vi "Partially Matched Crossover(PMX).vi"(10 "Ind 2":T1, 11 "Ind 1":T1) -> (2 "Child 2":T1, 3 "Child 1":T1)   [LabVIEW 2013, in "GA.lvclass"]
uses:
  GA.lvclass
  Controls/Solution_GA.ctl
panel:
  out "cxpoint2":i32
  out "cxpoint1":i32
  out "Child2 Schedule":u16[](array[numeric])
  out "Child 1 Schedule":u16[](array[numeric])
  out "p2":i32[](array[numeric])
  out "p1":i32[](array[numeric])
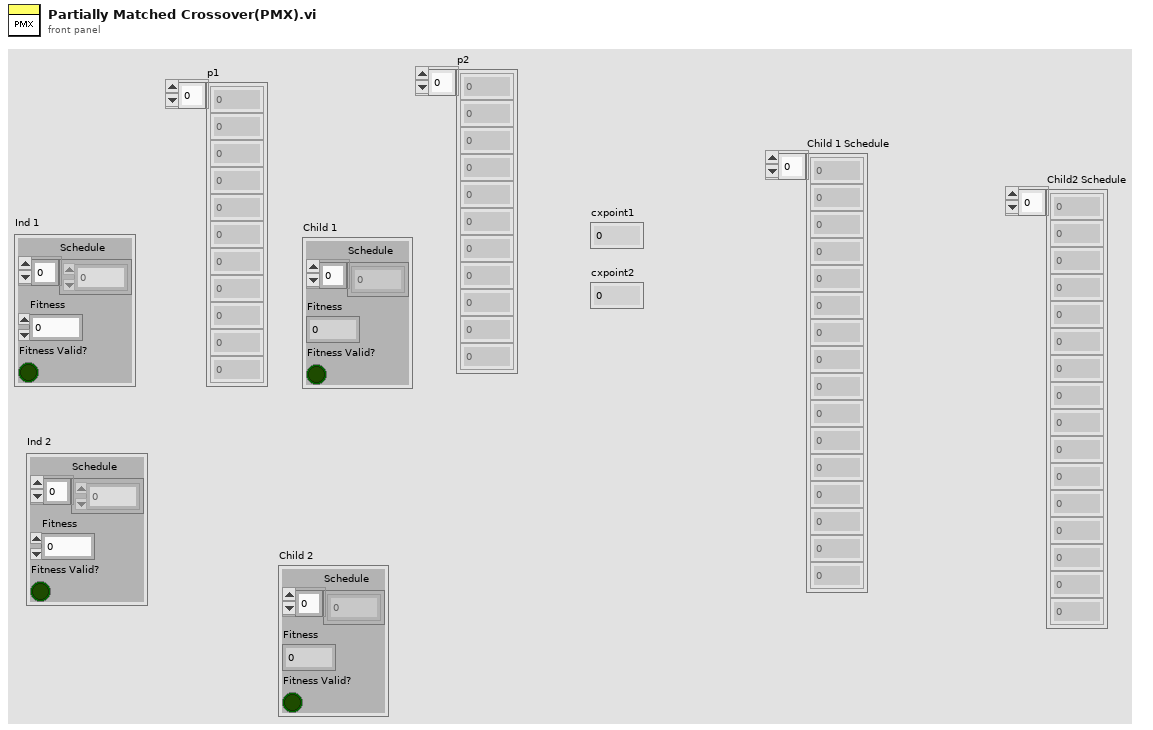
[diagram p1: front panel]
types:
  T1 = typedef "Solution_GA.ctl" = cluster{"Schedule":u16[], "Fitness":u16, "Fitness Valid?":bool}
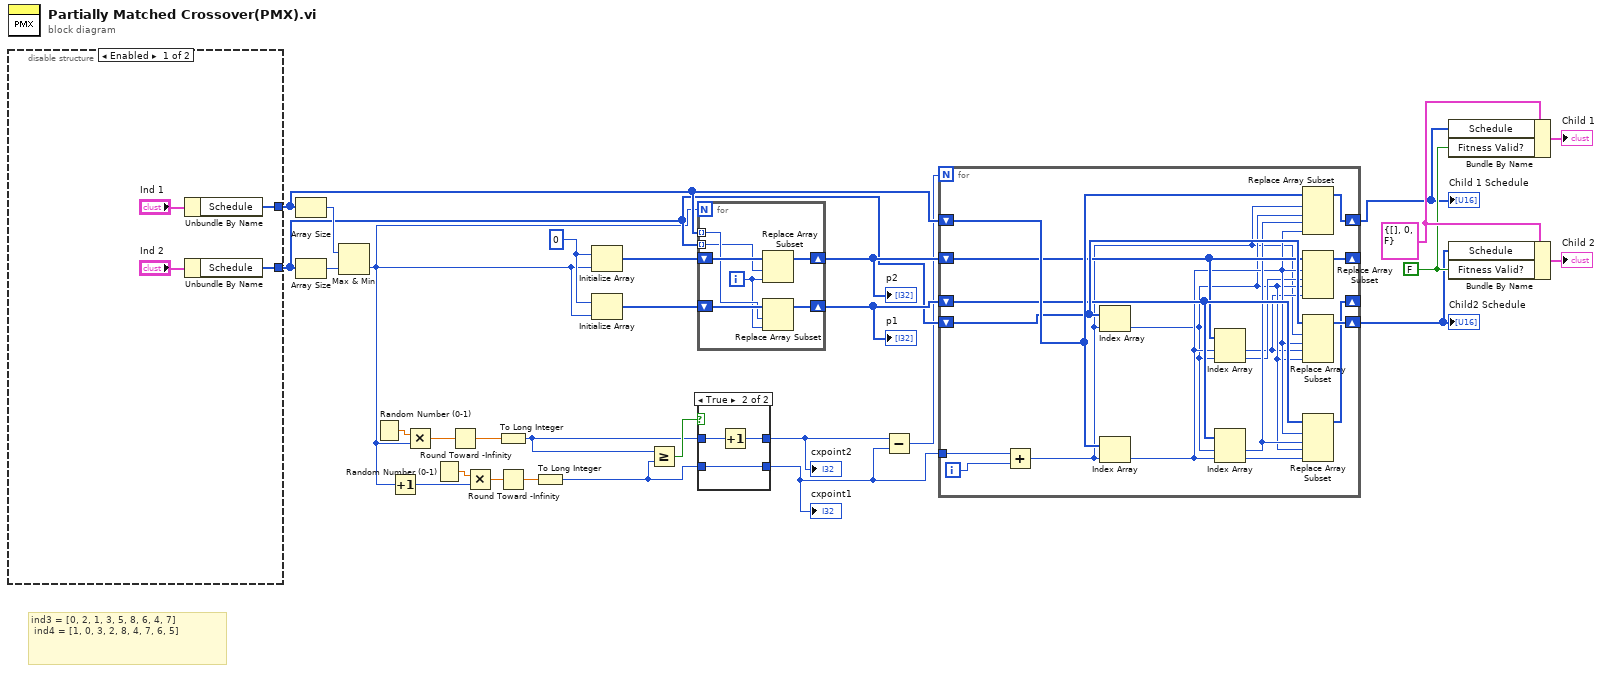
[diagram p0: block diagram]
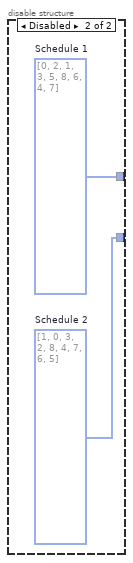
[diagram p3: hidden frame]
diagram:
  w21 = FALSE ("Fitness Valid?")
  w22 = T1 {"Schedule"=[], "Fitness"=0, "Fitness Valid?"=FALSE} ("Child 2")
  w27 = 0
  # "ind3 = [0, 2, 1, 3, 5, 8, 6, 4, 7]\n\tind4 = [1, 0, 3, 2, 8, 4, 7, 6, 5]"
  n1 = disable-structure shown="Enabled" {
    disable-tunnel: [w32 w35] -> w16
    disable-tunnel: [w30 w34] -> w15
    frame Enabled {
      n2 = Unbundle By Name("Ind 1") -> ("Schedule"=w32:u16[])
      n3 = Unbundle By Name("Ind 2") -> ("Schedule"=w30:u16[])
    }
    frame Disabled {
      w34 = u16[] [1, 0, 3, 2, 8, 4, 7, 6, 5]  # Schedule 2
      w35 = u16[] [0, 2, 1, 3, 5, 8, 6, 4, 7]  # Schedule 1
    }
  }
  n4 = Array Size(array=w16) -> (size(s)=w29:i32)
  n5 = Array Size(array=w15) -> (size(s)=w28:i32)
  n6 = Max & Min(x=w29, y=w28) -> (min(x,y)=w14:i32)  [unwired: 1 out]
  n7 = Random Number (0-1)() -> (number: 0 to 1=w6:dbl)
  n8 = Increment(x=w14) -> (x+1=w9:i32)
  n9 = Multiply(x=w6, y=w14) -> (x*y=w5:dbl)
  n10 = Random Number (0-1)() -> (number: 0 to 1=w10:dbl)
  n11 = Round Toward -Infinity(1:w5) -> (0:w4:dbl)
  n12 = Multiply(x=w10, y=w9) -> (x*y=w8:dbl)
  n13 = To Long Integer(number=w4) -> (32bit integer=w2:i32)
  n14 = Round Toward -Infinity(1:w8) -> (0:w7:dbl)
  n15 = To Long Integer(number=w7) -> (32bit integer=w1:i32)
  n16 = Initialize Array(w27, w14) -> (w25:i32[])
  n17 = Initialize Array(w27, w14) -> (w26:i32[])
  n18 = Greater Or Equal?(x=w2, y=w1) -> (x >= y?=w3:bool)
  n19 = for {
    N: w14 -> [_]
    tunnel: w16 -> [w40] mode=indexing
    tunnel: w15 -> [w39] mode=indexing
    shift-right: [w37] -> w24
    shift-left: w26 -> [w42]
    shift-right: [w36] -> w23
    shift-left: w25 -> [w41]
    i -> [w38]
    n20 = Replace Array Subset(array=w41, new element=w38, index=w39) -> (w36:i32[])
    n21 = Replace Array Subset(array=w42, new element=w38, index=w40) -> (w37:i32[])
  }
  "p1" <- w24
  "p2" <- w23
  n22 = case shown="True" w3 {
    tunnel: w2 -> [w44 w47]
    tunnel: [w43 w46] -> w11
    tunnel: w1 -> [w43 w45]
    tunnel: [w44 w45] -> w12
    frame False {
    }
    frame True {
      n23 = Increment(x=w47) -> (x+1=w46:i32)
    }
  }
  "cxpoint1" <- w12
  "cxpoint2" <- w11
  n24 = Subtract(x=w11, y=w12) -> (x-y=w13:i32)
  n25 = for {
    N: w13 -> [_]
    shift-right: [w60] -> w18
    shift-left: w16 -> [w64]
    shift-right: [w59] -> w17
    shift-left: w15 -> [w63]
    shift-right: [w58] -> _
    shift-left: w24 -> [w62]
    shift-right: [w57] -> _
    shift-left: w23 -> [w61]
    tunnel: w12 -> [w56]
    i -> [w49]
    n26 = Add(x=w56, y=w49) -> (x+y=w48:i32)
    n27 = Index Array(array=w63, index=w48) -> (element=w51:u16)
    n28 = Index Array(array=w64, index=w48) -> (element=w53:u16)
    n29 = Index Array(array=w61, index #1=w53, index #2=w51) -> (element #1=w50:i32, element #2=w52:i32)
    n30 = Index Array(array=w62, index #1=w51, index #2=w53) -> (element #1=w55:i32, element #2=w54:i32)
    n31 = Replace Array Subset(array=w64, new element #1=w51, index #1=w48, new element #2=w53, index #2=w55) -> (w60:u16[])
    n32 = Replace Array Subset(array=w61, new element #1=w52, index #1=w53, new element #2=w50, index #2=w51) -> (w57:i32[])
    n33 = Replace Array Subset(array=w63, new element #1=w53, index #1=w48, new element #2=w51, index #2=w50) -> (w59:u16[])
    n34 = Replace Array Subset(array=w62, new element #1=w55, index #1=w53, new element #2=w54, index #2=w51) -> (w58:i32[])
  }
  "Child 1 Schedule" <- w18
  "Child2 Schedule" <- w17
  n35 = Bundle By Name(cluster=w22, "Schedule"=w18, "Fitness Valid?"=w21) -> (→"Child 1":T1)
  n36 = Bundle By Name(cluster=w22, "Schedule"=w17, "Fitness Valid?"=w21) -> (→"Child 2":T1)
